vi "Text-to-speech Simple Example.vi"() -> ()   [LabVIEW 2012]
doc: "This VI demonstrates the use of each component in the SAPI.TTS library."
uses:
  SAPI TTS Library/SubVIs/SAPI_Speak_Text_String_SubVI.vi
  SAPI TTS Library/SAPI.TTS.lvlib
panel:
  in  "TTS Voice":u16(ring) items=["Microsoft Anna - English (United States)"]
  in  "Output Device":u16(ring) items=["Speakers (Realtek High Definition Audio)"]
  in  "Rate":i32(slide) min=-10 max=10 scale=-10.0..10.0
  in  "Volume":i32(slide)=100 min=0 max=100 scale=0.0..100.0
  out "Speaking...":bool
  in  "Text to speak":string="I want to eat an apple every day"
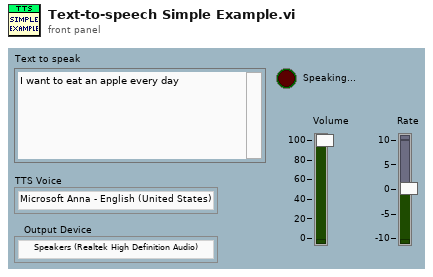
[diagram p1: front panel]
types:
  T1 = typedef "SAPI.TTS.lvlib/Speech object references.ctl" = cluster{"SpeechLib.ISpeechVoice":refnum<k7>, "GetVoices":refnum<k7>, "GetAudioOutputs":refnum<k7>}
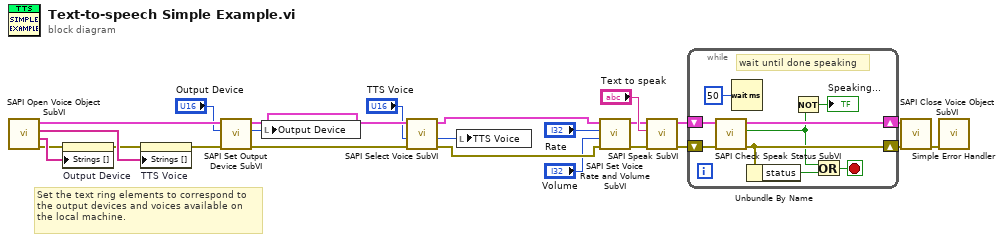
[diagram p0: block diagram]
diagram:
  # "Set the text ring elements to correspond to\nthe output devices and voices available on\nthe local machine."
  n1 = call "SAPI Open Voice Object SubVI.vi"() -> ("error out"=w13:errorcluster, "AudioOutputs"=w14:string[], "Voice Names"=w8:string[], "speech object references"=w12:T1)  [unwired: 8 in]
  n2 = property on="Output Device" class="Ring (strict)"(error in=w13, "Strings []"=w14) -> (error out=w5:errorcluster)  [unwired: 1 in, 1 out]
  n3 = property on="TTS Voice" class="Ring (strict)"(error in=w5, "Strings []"=w8) -> (error out=w4:errorcluster)  [unwired: 1 in, 1 out]
  n4 = call "SAPI Set Output Device SubVI.vi"("error in (no error)"=w4, "Device Number"="Output Device", "speech object references"=w12) -> ("error out"=w3:errorcluster, "Device Number"=w9:u16, "speech object references (out)"=w11:T1)  [unwired: 6 in]
  n5 = local write "Output Device"(w9) -> ()
  n6 = call "SAPI Select Voice SubVI.vi"("error in (no error)"=w3, "Voice Index (default voice: 0)"="TTS Voice", "speech object references"=w11) -> ("error out"=w18:errorcluster, "Voice Index (coerced)"=w6:u16, "speech object references (out)"=w20:T1)  [unwired: 6 in]
  n7 = local write "TTS Voice"(w6) -> ()
  n8 = call "SAPI Set Voice Rate and Volume SubVI.vi"("error in (no error)"=w18, "Volume (0 to 100: 100)"="Volume", "Speech Rate (-10 to 10: 0)"="Rate", "speech object references"=w20) -> ("error out"=w17:errorcluster, "speech object references (out)"=w19:T1)  [unwired: 6 in]
  n9 = call-poly "SAPI Speak SubVI.vi"("error in (no error)"=w17, "Text to speak"="Text to speak", "speech object references"=w19) -> ("error out"=w23:errorcluster, "speech object references (out)"=w24:T1)  [unwired: 7 in]
  n10 = while {
    shift-right: [w28] -> w1
    shift-left: w23 -> [w32]
    shift-right: [w29] -> w2
    shift-left: w24 -> [w33]
    stop <- w30 stop-if-true
    # "wait until done speaking"
    n11 = call "SAPI Check Speak Status SubVI.vi"("error in (no error)"=w32, "speech object references"=w33) -> ("error out"=w28:errorcluster, "Status (T: Done)"=w27:bool, "speech object references (out)"=w29:T1)  [unwired: 7 in]
    n12 = Wait (ms)(milliseconds to wait=u32 50) -> ()  [unwired: 1 out]
    n13 = Unbundle By Name(w28) -> ("status"=w31:bool)
    n14 = Not(x=w27) -> (.not. x?=→"Speaking...":bool)
    n15 = Or(x=w27, y=w31) -> (x .or. y?=w30:bool)
  }
  n16 = call "SAPI Close Voice Object SubVI.vi"("error in (no error)"=w1, "speech object references"=w2) -> ("error out"=w21:errorcluster)  [unwired: 9 in]
  n17 = call <vilib>:"Simple Error Handler.vi"("error in (no error)"=w21) -> ()  [unwired: 4 in, 5 out]
